vi "Substitute the assigned name for lib and lvclass.vi"(8 "error in":errorcluster, 10 "Project Name":string, 11 "Name to Lib Map":map{string, refnum<vi>}(c390)) -> (0 "error out":errorcluster, 3 "Name to Lib Map out":map{string, refnum<vi>}(c390))   [LabVIEW 2023, in "Plugin Generator.lvlib"]
uses:
  Plugin Generator.lvlib
  <vilib>/dlg_ctls.llb/Space Constant.vi
  <vilib>/Utility/EditLVLibs/Edit LVLibs.lvlib
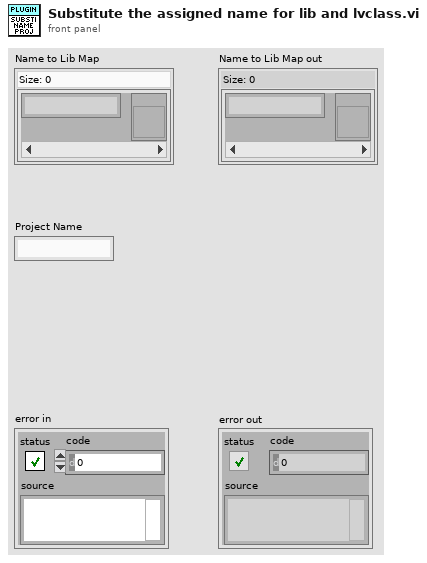
[diagram p1: front panel]
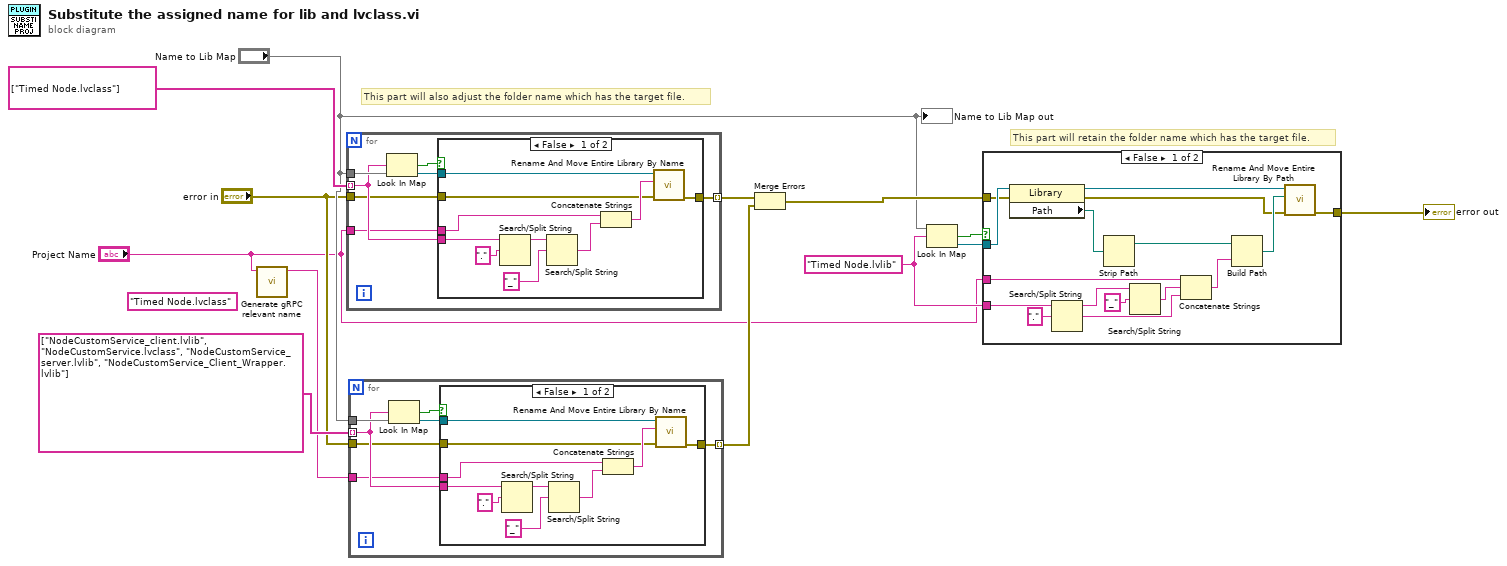
[diagram p0: block diagram]
diagram:
  (unwired) "Timed Node.lvclass" ("String")
  w13 = "Timed Node.lvlib" ("String")
  # "This part will retain the folder name which has the target file."
  # "This part will also adjust the folder name which has the target file."
  n1 = call "Generate gRPC relevant name.vi"("Project Name"="Project Name") -> ("gRPC Service Name"=w1:string)  [unwired: 9 in, 1 out]
  n2 = for {
    tunnel: string[] ["Timed Node.lvclass"] -> [w18] mode=indexing
    tunnel: "Name to Lib Map" -> [w20]
    tunnel: [w17] -> w9 mode=indexing
    tunnel: "Project Name" -> [w15]
    tunnel: "error in" -> [w14]
    n3 = Look In Map(map=w20, key=w18) -> (key not found?=w19:bool, value=w16:refnum<vi>)  [unwired: 1 in]
    n4 = case shown="False" w19 {
      tunnel: w18 -> [w28 _]
      tunnel: [w25 w31] -> w17
      tunnel: w16 -> [w23 _]
      tunnel: w15 -> [w22 _]
      tunnel: w14 -> [w21 w31]
      frame False {
        n5 = Search/Split String(string=w28, search string/char (-)=".") -> (substring before match=w26:string)  [unwired: 1 in, 2 out]
        n6 = Search/Split String(string=w26, search string/char (-)="_" ("regular expression")) -> (match + rest of string=w29:string)  [unwired: 1 in, 2 out]
        n7 = Concatenate Strings(w22, w29) -> (w24:string)
        n8 = call <vilib>:"Rename And Move Entire Library By Name.vi"("error in (no error)"=w21, "New name without file extension"=w24, "Library ref in"=w23) -> ("error out"=w25:errorcluster)  [unwired: 6 in, 2 out]
      }
      frame True {
      }
    }
  }
  n9 = for {
    tunnel: string[] ["NodeCustomService_client.lvlib", "NodeCustomService.lvclass", "NodeCustomService_server.lvlib", "NodeCustomService_Client_Wrapper.lvlib"] -> [w36] mode=indexing
    tunnel: "Name to Lib Map" -> [w38]
    tunnel: [w35] -> w3 mode=indexing
    tunnel: w1 -> [w33]
    tunnel: "error in" -> [w32]
    n10 = Look In Map(map=w38, key=w36) -> (key not found?=w37:bool, value=w34:refnum<vi>)  [unwired: 1 in]
    n11 = case shown="False" w37 {
      tunnel: w36 -> [w46 _]
      tunnel: [w43 w49] -> w35
      tunnel: w34 -> [w41 _]
      tunnel: w33 -> [w40 _]
      tunnel: w32 -> [w39 w49]
      frame False {
        n12 = Search/Split String(string=w46, search string/char (-)=".") -> (substring before match=w44:string)  [unwired: 1 in, 2 out]
        n13 = Search/Split String(string=w44, search string/char (-)="_" ("regular expression")) -> (match + rest of string=w47:string)  [unwired: 1 in, 2 out]
        n14 = Concatenate Strings(w40, w47) -> (w42:string)
        n15 = call <vilib>:"Rename And Move Entire Library By Name.vi"("error in (no error)"=w39, "New name without file extension"=w42, "Library ref in"=w41) -> ("error out"=w43:errorcluster)  [unwired: 6 in, 2 out]
      }
      frame True {
      }
    }
  }
  n16 = Merge Errors(w9, w3) -> (w7:errorcluster)
  n17 = Look In Map(map="Name to Lib Map", key=w13) -> (key not found?=w11:bool, value=w12:refnum<vi>)  [unwired: 1 in]
  n18 = case shown="False" w11 {
    tunnel: w12 -> [w53 _]
    tunnel: w13 -> [w61 _]
    tunnel: [w54 w66] -> w8
    tunnel: "Project Name" -> [w52 _]
    tunnel: w7 -> [w51 w66]
    frame False {
      n19 = property class="Library"(reference=w53, error in=w51) -> (reference out=w56:refnum<vi>, error out=w50:errorcluster, "Path"=w63:path)
      n20 = Search/Split String(string=w61, search string/char (-)=".") -> (substring before match=w59:string, match + rest of string=w57:string)  [unwired: 1 in, 1 out]
      n21 = Strip Path(path=w63) -> (stripped path=w62:path)  [unwired: 1 out]
      n22 = Search/Split String(string=w59, search string/char (-)="_" ("regular expression")) -> (match + rest of string=w64:string)  [unwired: 1 in, 2 out]
      n23 = Concatenate Strings(w52, w64, w57) -> (w58:string)
      n24 = Build Path(base path=w62, name or relative path=w58) -> (appended path=w55:path)
      n25 = call <vilib>:"Rename And Move Entire Library By Path.vi"("error in (no error)"=w50, "New library path"=w55, "Library ref in"=w56) -> ("error out"=w54:errorcluster)  [unwired: 7 in, 1 out]
    }
    frame True {
    }
  }
  "error out" <- w8
  "Name to Lib Map out" <- "Name to Lib Map"
